vi "PI_GCS3_Configuration_Setup_CSV.vi"(0 "System no.":i32=1 min=1 step=1, 5 "error in":errorcluster) -> (19 "error out":errorcluster)   [LabVIEW 2020]
doc: "Select axes which drive state is not \"Open\" and waits until enabled with EAX.\n\nWarning: Do not use this VI outside the GCS 3.0 Configuration Setup."
panel:
  # "Require GCS 3.0 standard on controller.\n\nWarning: Do not use this VI outside the\nGCS 3.0 Configuration Setup."
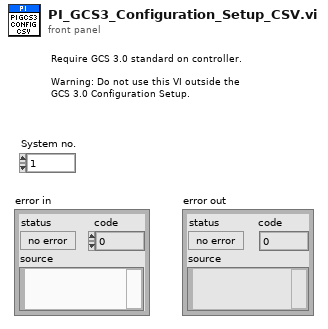
[diagram p1: front panel]
types:
  T1 = typedef "Syntax.ctl" = enum16{"GCS 1.0", "GCS 2.0", "GCS 3.0"}
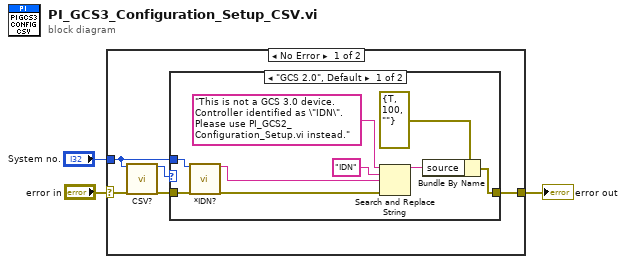
[diagram p0: block diagram]
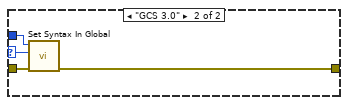
[diagram p2: hidden frame]
diagram:
  n1 = case shown="No Error" "error in" {
    selector: "error in" -> [w8 w22]
    tunnel: [w5 w22] -> w2
    tunnel: "System no." -> [w4 _]
    frame No Error {
      n2 = call "CSV?.vi"("System no."=w4, "error in"=w8) -> ("Syntax"=w6:T1, "error out"=w7:errorcluster)  [unwired: 16 in]
      n3 = case shown="\"GCS 2.0\", Default" w6 {
        selector: w6 -> [_ w18]
        tunnel: [w9 w19] -> w5
        tunnel: w7 -> [w14 w21]
        tunnel: w4 -> [w15 w20]
        frame "GCS 2.0", Default {
          n4 = call "*IDN?.vi"("System no."=w15, "error in"=w14) -> ("Identification"=w12:string, "error out"=w13:errorcluster)  [unwired: 16 in]
          n5 = Search and Replace String(input string="This is not a GCS 3.0 device. Controller identified as \"IDN\". Please use PI_GCS2_Configuration_Setup.vi instead." ("source"), search string="IDN", replace string=w12, error in=w13) -> (result string=w10:string)  [unwired: 4 in, 3 out]
          n6 = Bundle By Name(cluster=errorcluster {"status"=TRUE, "code"=100, "source"=""} ("error in"), "source"=w10) -> (w9:errorcluster)
        }
        frame "GCS 3.0" {
          n7 = call "Set Syntax In Global.vi"("error in"=w21, "Syntax"=w18, "System no."=w20) -> ("error out"=w19:errorcluster)  [unwired: 8 in]
        }
      }
    }
    frame Error {
    }
  }
  "error out" <- w2
